vi "Lifter_Main_Vi.vi"() -> ()   [LabVIEW 2019]
panel:
  out "ADC":dbl(slide) scale=59000.0..-200.0
  in  "address":string="192.168.24.142"
  out "error IO":errorcluster
  out "Status":bool
  out "Motor Status":string
  out "ADC error out 3":errorcluster
  out "ADC Voltage":dbl format="%.4f"
  in  "error in":errorcluster
  in  "Down 100":bool
  in  "Up 100":bool
  out "TCP error out":errorcluster
  in  "Steps":i32
  in  "Down":bool
  in  "Up":bool
  out "Possition":i32(slide) scale=59000.0..-200.0
  in  "Reset":bool
  out "Lower Limit":bool
  out "Upper Limmit":bool
  out "Top":bool
  out "Middle":bool
  out "Bottom":bool
  out "Anneal":bool
  out "Home":bool
  in  "stop":bool
  out "Position Count":dbl
  in  "Cup Position":T1(ring)
  out "Loop Running":bool
  in  "stop2":bool
  in  "remote port":u16=7776
  in  "Move":bool
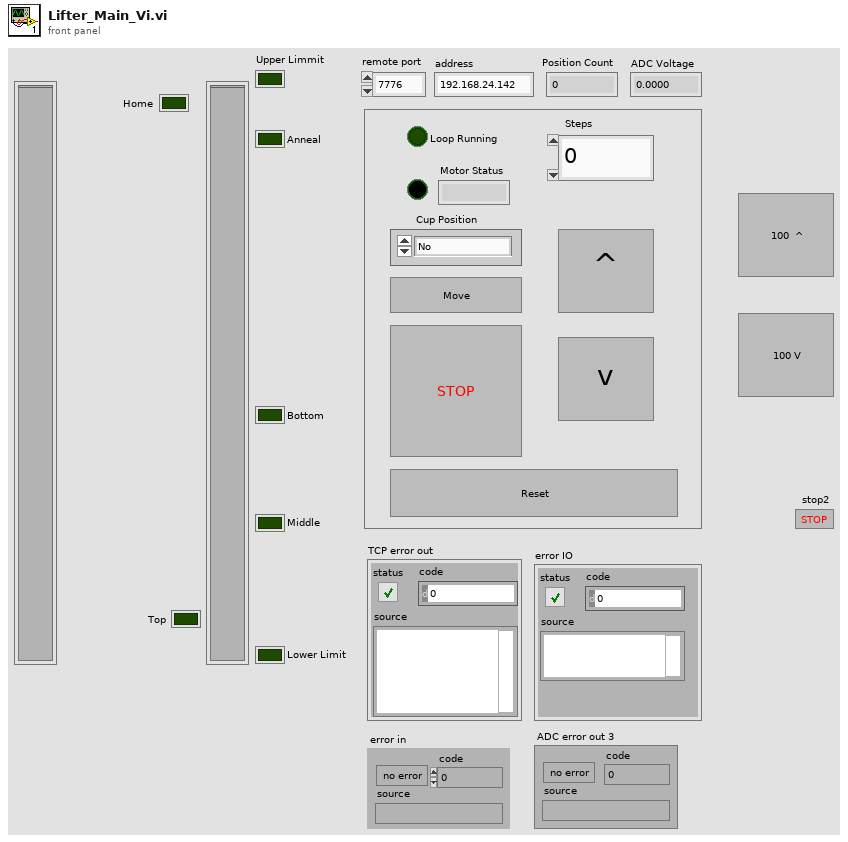
[diagram p1: front panel]
types:
  T1 = enum16{"No", "Home", "Anneal", "Bottom Cup", "Middle Cup", "Top Cup"}
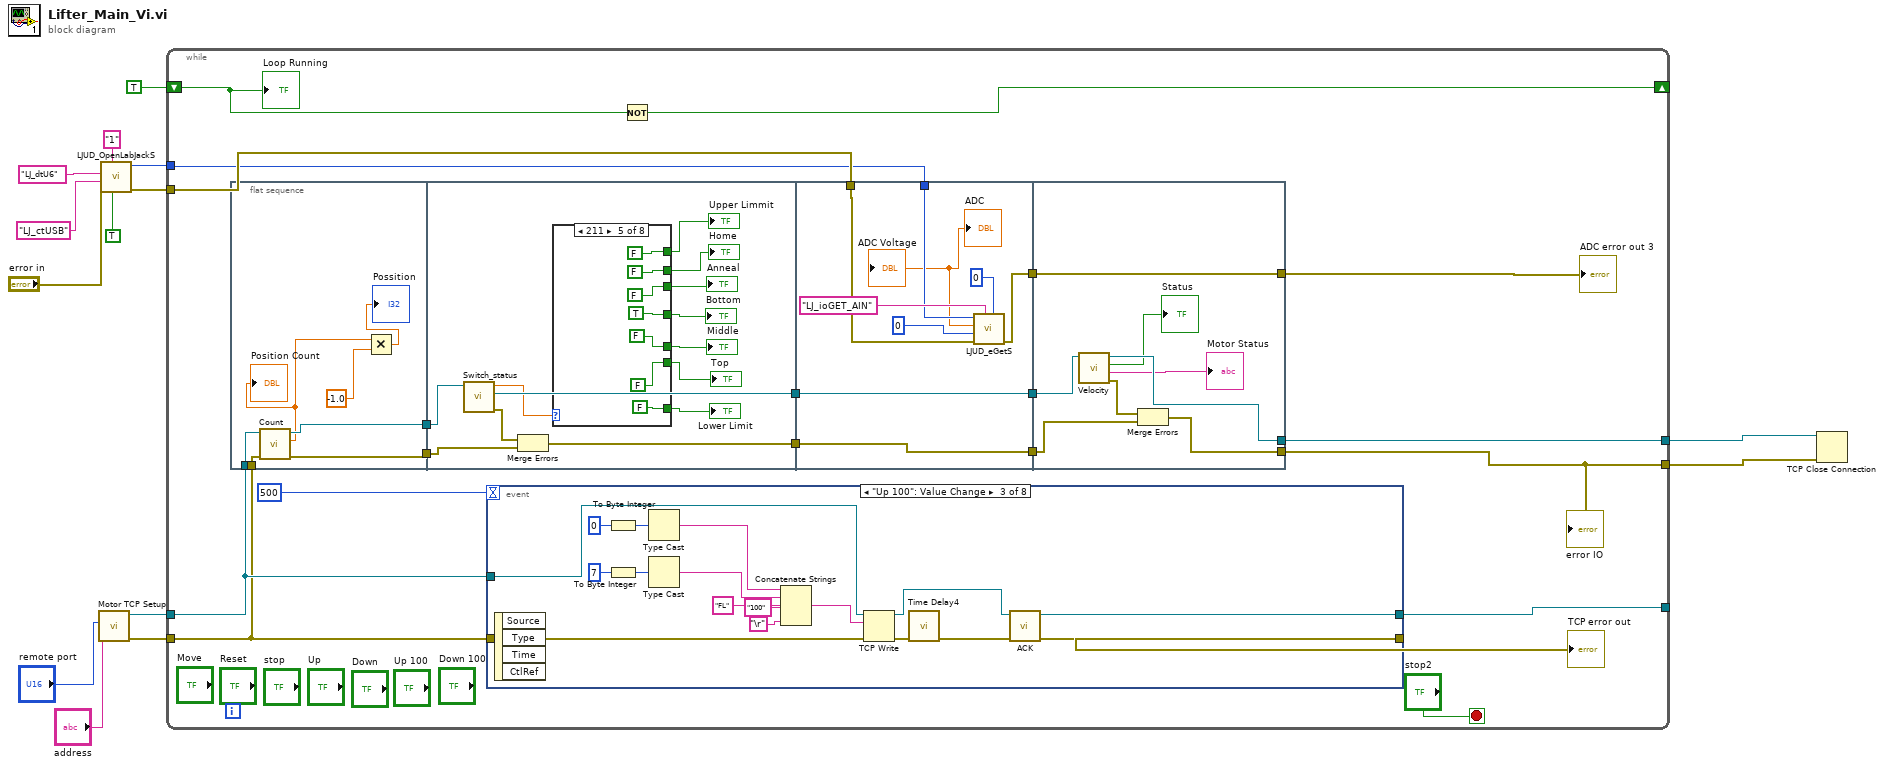
[diagram p0: block diagram]
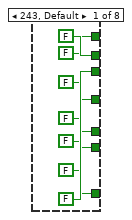
[diagram p2: hidden frame]
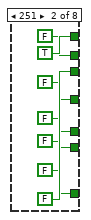
[diagram p3: hidden frame]
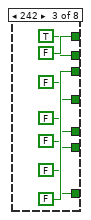
[diagram p4: hidden frame]
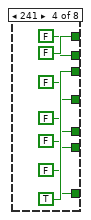
[diagram p5: hidden frame]
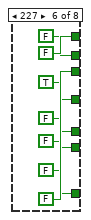
[diagram p6: hidden frame]
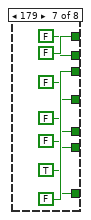
[diagram p7: hidden frame]
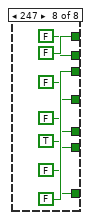
[diagram p8: hidden frame]
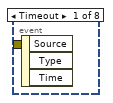
[diagram p9: hidden frame]
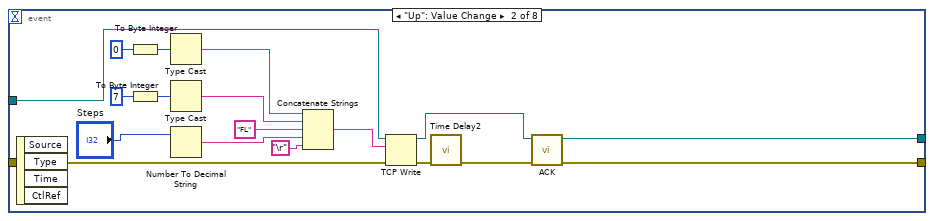
[diagram p10: hidden frame]
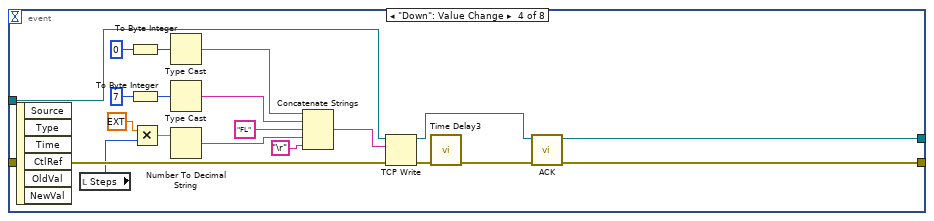
[diagram p11: hidden frame]
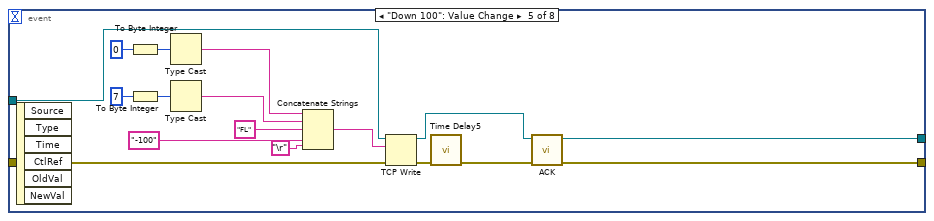
[diagram p12: hidden frame]
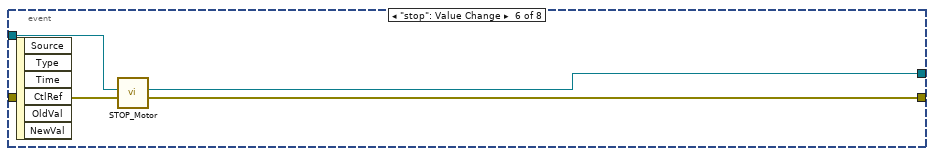
[diagram p13: hidden frame]
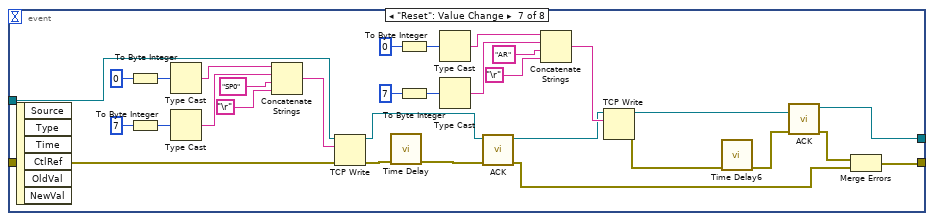
[diagram p14: hidden frame]
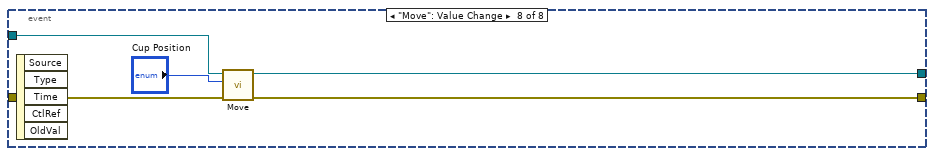
[diagram p15: hidden frame]
diagram:
  n1 = call "Motor TCP Setup.vi"("address"="address", "remote port or service name"="remote port") -> ("error out"=w13:errorcluster, "TCP Network Connection out"=w12:refnum<k5>)  [unwired: 8 in]
  n2 = call <vilib>:"LJUD_OpenLabJackS.vi"("FirstFound"=TRUE, "Address"="1", "error in"="error in", "ConnectionType"="LJ_ctUSB", "DeviceType"="LJ_dtU6") -> ("error out"=w4:errorcluster, "Handle"=w3:i32)  [unwired: 4 in, 1 out]
  n3 = while {
    shift-right: [w32] -> _
    shift-left: TRUE ("Boolean") -> [w33]
    tunnel: w13 -> [w28]
    tunnel: w12 -> [w29]
    tunnel: [w31] -> _
    tunnel: [w25] -> w10
    tunnel: w4 -> [w22]
    tunnel: w3 -> [w21]
    tunnel: [w16] -> w2
    stop <- "stop2" stop-if-true
    n4 = flat-sequence {
      tunnel: w29 -> [w41]
      tunnel: w28 -> [w40]
      tunnel: [w39] -> w27
      tunnel: [w38] -> w26
      tunnel: w27 -> [w54]
      tunnel: w26 -> [w51]
      tunnel: [w53] -> w24
      tunnel: [w50] -> w23
      tunnel: w24 -> [w119]
      tunnel: w23 -> [w118]
      tunnel: w22 -> [w115]
      tunnel: w21 -> [w113]
      tunnel: [w119] -> w19
      tunnel: [w118] -> w18
      tunnel: [w112] -> w17
      tunnel: [w127] -> w20
      tunnel: [w125] -> w25
      tunnel: w19 -> [w120]
      tunnel: w18 -> [w126]
      tunnel: w17 -> [w127]
      tunnel: [w124] -> w16
      frame #0 {
        n5 = call "Count.vi"("error in (no error)"=w40, "TCP Network Connection in"=w41) -> ("error out"=w38:errorcluster, "Position Count"=w37:dbl, "TCP Network Connection out"=w39:refnum<k5>)  [unwired: 7 in]
        "Position Count" <- w37
        n6 = Multiply(x=w37, y=-1.0) -> (x*y=→"Possition":dbl)
      }
      frame #1 {
        n7 = call "Switch_status.vi"("TCP Network Connection in"=w54) -> ("error out"=w52:errorcluster, "TCP Network Connection out"=w53:refnum<k5>, "Numeric"=w49:dbl)  [unwired: 8 in]
        n8 = Merge Errors(w52, w51) -> (w50:errorcluster)
        n9 = case shown="211" w49 {
          tunnel: [FALSE ("Home") FALSE ("Home") TRUE ("Home") FALSE ("Home") FALSE ("Home") FALSE ("Home") FALSE ("Home") FALSE ("Home")] -> w42
          tunnel: [FALSE ("Home") FALSE ("Home") FALSE ("Home") TRUE ("Home") FALSE ("Home") FALSE ("Home") FALSE ("Home") FALSE ("Home")] -> w43
          tunnel: [FALSE ("Home") FALSE ("Home") FALSE ("Home") FALSE ("Home") TRUE ("Home") FALSE ("Home") FALSE ("Home") FALSE ("Home")] -> w44
          tunnel: [FALSE ("Home") FALSE ("Home") FALSE ("Home") FALSE ("Home") FALSE ("Home") TRUE ("Home") FALSE ("Home") FALSE ("Home")] -> w45
          tunnel: [FALSE ("Home") FALSE ("Home") FALSE ("Home") FALSE ("Home") FALSE ("Home") FALSE ("Home") TRUE ("Home") FALSE ("Home")] -> w46
          tunnel: [FALSE ("Home") TRUE ("Home") FALSE ("Home") FALSE ("Home") FALSE ("Home") FALSE ("Home") FALSE ("Home") FALSE ("Home")] -> w47
          tunnel: [FALSE ("Home") FALSE ("Home") FALSE ("Home") FALSE ("Home") FALSE ("Home") FALSE ("Home") FALSE ("Home") TRUE ("Home")] -> w48
          frame 243, Default {
          }
          frame 251 {
          }
          frame 242 {
          }
          frame 241 {
          }
          frame 211 {
          }
          frame 227 {
          }
          frame 179 {
          }
          frame 247 {
          }
        }
        "Home" <- w42
        "Anneal" <- w43
        "Bottom" <- w44
        "Middle" <- w45
        "Top" <- w46
        "Upper Limmit" <- w47
        "Lower Limit" <- w48
      }
      frame #2 {
        n10 = call <vilib>:"LJUD_eGetS.vi"("Channel"=0, "IOType"="LJ_ioGET_AIN", "error in"=w115, "x1"=0, "Handle In"=w113) -> ("error out"=w112:errorcluster, "Value Read"=→"ADC Voltage" →"ADC":dbl)  [unwired: 4 in, 1 out]
      }
      frame #3 {
        n11 = call "Velocity.vi"("connection ID"=w120) -> ("connection ID out"=w124:refnum<k5>, "Status"=→"Status":bool, "Motor Status"=→"Motor Status":string, "error out"=w123:errorcluster)  [unwired: 6 in]
        n12 = Merge Errors(w123, w126) -> (w125:errorcluster)
      }
    }
    n13 = event shown="[2] \"Up 100\": Value Change" {
      selector: _ -> [_ _ _ _ _ _ _ _]
      dyn-events: _ -> [_ _ _ _ _ _ _ _]
      timeout: 500 -> [_ _ _ _ _ _ _ _]
      tunnel: w28 -> [_ w130 w148 w167 w185 w203 w225 w238]
      tunnel: w29 -> [_ w129 w147 w166 w184 w202 w224 w237]
      tunnel: [_ w134 w152 w168 w186 w201 w207 w236] -> w31
      tunnel: [_ w135 w153 w169 w187 w200 w205 w235] -> w15
      event Timeout {
        n14 = event-data() -> ()  [unwired: 1 in, 3 out]
      }
      event "Up": Value Change {
        n15 = event-data() -> ()  [unwired: 1 in, 4 out]
        n16 = To Byte Integer(number=i8 0) -> (8bit integer=w139:i8)
        n17 = To Byte Integer(number=i8 7) -> (8bit integer=w142:i8)
        n18 = Type Cast(x=w139) -> (*(type *) &x=w140:string)  [unwired: 1 in]
        n19 = Type Cast(x=w142) -> (*(type *) &x=w141:string)  [unwired: 1 in]
        n20 = Number To Decimal String(number="Steps") -> (decimal integer string=w144:string)  [unwired: 1 in]
        n21 = Concatenate Strings(w140, w141, "FL" ("string"), w144, "\r") -> (w136:string)
        n22 = TCP Write(connection ID=w129, data in=w136, error in (no error)=w130) -> (connection ID out=w133:refnum<k5>, error out=w132:errorcluster)  [unwired: 1 in, 1 out]
        n23 = call "Time Delay2"("error in (no error)"=w132) -> ("error out"=w131:errorcluster)  [unwired: 10 in]
        n24 = call "ACK.vi"("error in (no error)"=w131, "TCP Network Connection in"=w133) -> ("error out"=w135:errorcluster, "TCP Network Connection out"=w134:refnum<k5>)  [unwired: 7 in, 1 out]
      }
      event "Up 100": Value Change {
        n25 = event-data() -> ()  [unwired: 1 in, 4 out]
        n26 = To Byte Integer(number=i8 0) -> (8bit integer=w157:i8)
        n27 = To Byte Integer(number=i8 7) -> (8bit integer=w160:i8)
        n28 = Type Cast(x=w157) -> (*(type *) &x=w158:string)  [unwired: 1 in]
        n29 = Type Cast(x=w160) -> (*(type *) &x=w159:string)  [unwired: 1 in]
        n30 = Concatenate Strings(w158, w159, "FL" ("string"), "100" ("string"), "\r") -> (w154:string)
        n31 = TCP Write(connection ID=w147, data in=w154, error in (no error)=w148) -> (connection ID out=w151:refnum<k5>, error out=w150:errorcluster)  [unwired: 1 in, 1 out]
        n32 = call "Time Delay4"("error in (no error)"=w150) -> ("error out"=w149:errorcluster)  [unwired: 10 in]
        n33 = call "ACK.vi"("error in (no error)"=w149, "TCP Network Connection in"=w151) -> ("error out"=w153:errorcluster, "TCP Network Connection out"=w152:refnum<k5>)  [unwired: 7 in, 1 out]
      }
      event "Down": Value Change {
        n34 = event-data() -> ()  [unwired: 1 in, 6 out]
        n35 = local read "Steps"() -> (w163:i32)
        n36 = To Byte Integer(number=i8 0) -> (8bit integer=w176:i8)
        n37 = To Byte Integer(number=i8 7) -> (8bit integer=w179:i8)
        n38 = Multiply(x=ext -1.0, y=w163) -> (x*y=w164:ext)
        n39 = Type Cast(x=w176) -> (*(type *) &x=w177:string)  [unwired: 1 in]
        n40 = Type Cast(x=w179) -> (*(type *) &x=w178:string)  [unwired: 1 in]
        n41 = Number To Decimal String(number=w164) -> (decimal integer string=w181:string)  [unwired: 1 in]
        n42 = Concatenate Strings(w177, w178, "FL" ("string"), w181, "\r") -> (w173:string)
        n43 = TCP Write(connection ID=w166, data in=w173, error in (no error)=w167) -> (connection ID out=w172:refnum<k5>, error out=w171:errorcluster)  [unwired: 1 in, 1 out]
        n44 = call "Time Delay3"("error in (no error)"=w171) -> ("error out"=w170:errorcluster)  [unwired: 10 in]
        n45 = call "ACK.vi"("error in (no error)"=w170, "TCP Network Connection in"=w172) -> ("error out"=w169:errorcluster, "TCP Network Connection out"=w168:refnum<k5>)  [unwired: 7 in, 1 out]
      }
      event "Down 100": Value Change {
        n46 = event-data() -> ()  [unwired: 1 in, 6 out]
        n47 = To Byte Integer(number=i8 0) -> (8bit integer=w194:i8)
        n48 = To Byte Integer(number=i8 7) -> (8bit integer=w197:i8)
        n49 = Type Cast(x=w194) -> (*(type *) &x=w195:string)  [unwired: 1 in]
        n50 = Type Cast(x=w197) -> (*(type *) &x=w196:string)  [unwired: 1 in]
        n51 = Concatenate Strings(w195, w196, "FL" ("string"), "-100" ("string"), "\r") -> (w191:string)
        n52 = TCP Write(connection ID=w184, data in=w191, error in (no error)=w185) -> (connection ID out=w190:refnum<k5>, error out=w189:errorcluster)  [unwired: 1 in, 1 out]
        n53 = call "Time Delay5"("error in (no error)"=w189) -> ("error out"=w188:errorcluster)  [unwired: 10 in]
        n54 = call "ACK.vi"("error in (no error)"=w188, "TCP Network Connection in"=w190) -> ("error out"=w187:errorcluster, "TCP Network Connection out"=w186:refnum<k5>)  [unwired: 7 in, 1 out]
      }
      event "stop": Value Change {
        n55 = event-data() -> ()  [unwired: 1 in, 6 out]
        n56 = call "STOP_Motor.vi"("error in (no error)"=w203, "TCP Network Connection in"=w202) -> ("error out"=w200:errorcluster, "TCP Network Connection out"=w201:refnum<k5>)  [unwired: 8 in]
      }
      event "Reset": Value Change {
        n57 = event-data() -> ()  [unwired: 1 in, 6 out]
        n58 = To Byte Integer(number=i8 0) -> (8bit integer=w233:i8)
        n59 = To Byte Integer(number=i8 7) -> (8bit integer=w234:i8)
        n60 = Type Cast(x=w233) -> (*(type *) &x=w227:string)  [unwired: 1 in]
        n61 = Type Cast(x=w234) -> (*(type *) &x=w228:string)  [unwired: 1 in]
        n62 = Concatenate Strings(w227, w228, "SP0" ("string"), "\r") -> (w230:string)
        n63 = TCP Write(connection ID=w224, data in=w230, error in (no error)=w225) -> (connection ID out=w223:refnum<k5>, error out=w222:errorcluster)  [unwired: 1 in, 1 out]
        n64 = call "Time Delay"("error in (no error)"=w222) -> ("error out"=w221:errorcluster)  [unwired: 10 in]
        n65 = To Byte Integer(number=i8 0) -> (8bit integer=w219:i8)
        n66 = To Byte Integer(number=i8 7) -> (8bit integer=w220:i8)
        n67 = Type Cast(x=w219) -> (*(type *) &x=w213:string)  [unwired: 1 in]
        n68 = Type Cast(x=w220) -> (*(type *) &x=w214:string)  [unwired: 1 in]
        n69 = call "ACK.vi"("error in (no error)"=w221, "TCP Network Connection in"=w223) -> ("error out"=w204:errorcluster, "TCP Network Connection out"=w211:refnum<k5>)  [unwired: 7 in, 1 out]
        n70 = Concatenate Strings(w213, w214, "AR" ("string"), "\r") -> (w216:string)
        n71 = TCP Write(connection ID=w211, data in=w216) -> (connection ID out=w208:refnum<k5>, error out=w210:errorcluster)  [unwired: 2 in, 1 out]
        n72 = call "Time Delay6"("error in (no error)"=w210) -> ("error out"=w209:errorcluster)  [unwired: 10 in]
        n73 = call "ACK.vi"("error in (no error)"=w209, "TCP Network Connection in"=w208) -> ("error out"=w206:errorcluster, "TCP Network Connection out"=w207:refnum<k5>)  [unwired: 7 in, 1 out]
        n74 = Merge Errors(w206, w204) -> (w205:errorcluster)
      }
      event "Move": Value Change {
        n75 = event-data() -> ()  [unwired: 1 in, 5 out]
        n76 = call "Move.vi"("error in (no error)"=w238, "Cup Position"="Cup Position", "TCP Network Connection in"=w237) -> ("error out"=w235:errorcluster, "TCP Network Connection out"=w236:refnum<k5>)  [unwired: 6 in, 1 out]
      }
    }
    "TCP error out" <- w15
    n77 = Not(x=w33) -> (.not. x?=w32:bool)
    "Loop Running" <- w33
    "ADC error out 3" <- w20
    "error IO" <- w25
  }
  n78 = TCP Close Connection(connection ID=w2, error in (no error)=w10) -> ()  [unwired: 1 in, 2 out]
